vi "user_input.vi"() -> ()   [LabVIEW 2017]
uses:
  controls/AccountCmd.ctl
  controls/UpdateMessageCmd.ctl
  controls/UpdateMessageCtl.ctl
  controls/UserInputStateCmd.ctl
  controls/DisplayCommanda.ctl
  Downloads/ATM Simulator/Controls/DisplayControl.ctl
panel:
  out "queue 2":refnum<queue>
  in  "queue":refnum<queue>
  out "Parcel number":string
  in  "Phone number":string
  in  "Parcel number":string
  in  "User Input State":T1
  out "error out":errorcluster
  in  "error in (no error)":errorcluster
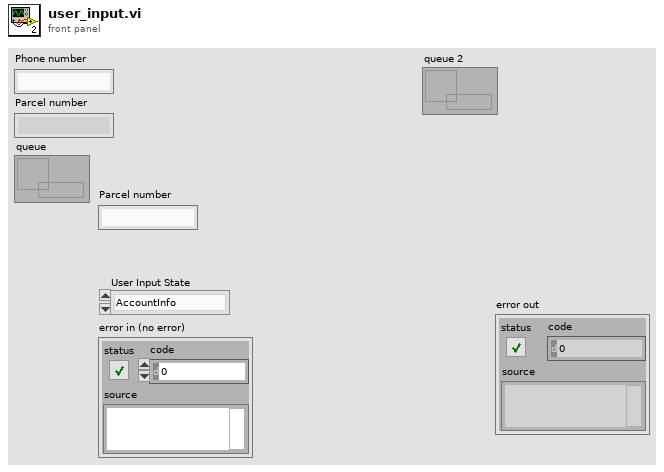
[diagram p1: front panel]
types:
  T1 = typedef "UserInputStateCmd.ctl" = enum16{"AccountInfo", "Withdrawal", "Deposit"}
  T2 = typedef "AccountCmd.ctl" = enum16{"Get parcel", "Get number", "Deposit", "Withdrawal"}
  T3 = typedef "UpdateMessageCtl.ctl" = cluster{"Command":T4, "Data":variant}
  T4 = typedef "UpdateMessageCmd.ctl" = enum16{"Welcome", "Main Menu", "Account Failed", "Session Terminated", "Deposit", "Deposit Complete", "Withdrawal", "Withdrawal Complete"}
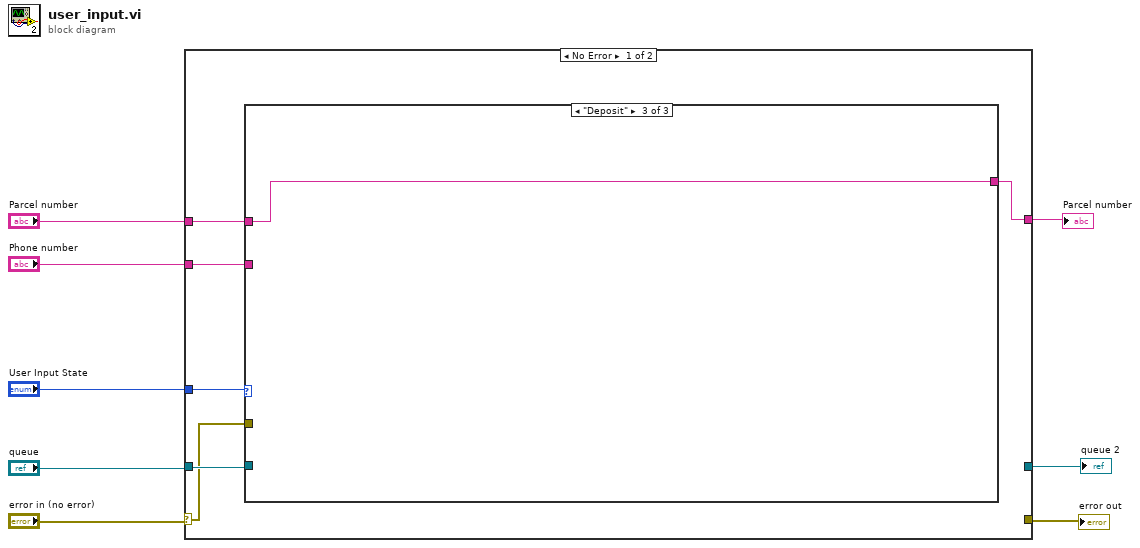
[diagram p0: block diagram]
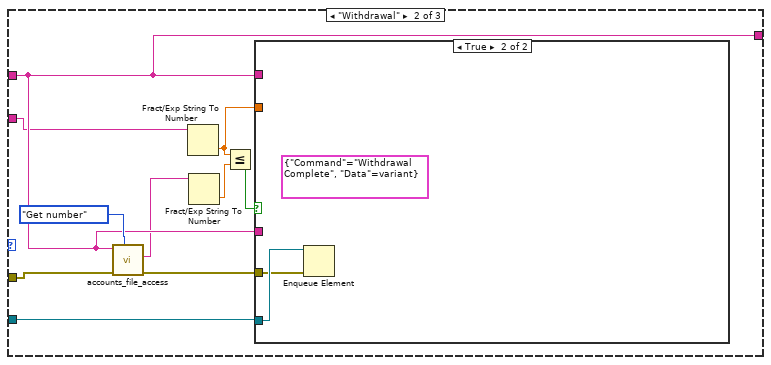
[diagram p3: hidden frame]
diagram:
  n1 = case shown="No Error" "error in (no error)" {
    selector: "error in (no error)" -> [w13 w31]
    tunnel: "queue" -> [w14 w30]
    tunnel: "User Input State" -> [w12 _]
    tunnel: "Parcel number" -> [w11 w29]
    tunnel: "Phone number" -> [w10 _]
    tunnel: [w9 w29] -> w3
    tunnel: [_ w31] -> w2
    tunnel: [_ w30] -> w1
    frame No Error {
      n2 = case shown="\"Deposit\"" w12 {
        tunnel: w14 -> [_ w25 _]
        tunnel: w13 -> [_ w22 _]
        tunnel: w11 -> [w15 w23 w28]
        tunnel: w10 -> [_ w19 _]
        tunnel: [w15 w23 w28] -> w9
        frame "AccountInfo", Default {
        }
        frame "Withdrawal" {
          n3 = call "accounts_file_access.vi"("AccountCommand"=AccountCmd."Get number", "error in (no error)"=w22, "Account"=w23) -> ("error out"=w21:errorcluster, "Value Out"=w20:string)  [unwired: 6 in]
          n4 = Fract/Exp String To Number(string=w19) -> (number=w18:dbl)  [unwired: 3 in, 1 out]
          n5 = Fract/Exp String To Number(string=w20) -> (number=w17:dbl)  [unwired: 3 in, 1 out]
          n6 = Less Or Equal?(x=w18, y=w17) -> (x <= y?=w16:bool)
          n7 = case shown="True" w16 {
            tunnel: w25 -> [_ w27]
            tunnel: w23 -> [_ _]
            tunnel: w23 -> [_ _]
            tunnel: w21 -> [_ w26]
            tunnel: w18 -> [_ _]
            frame False {
            }
            frame True {
              (unwired) T3 {"Command"=enum."Withdrawal Complete", "Data"=variant} ("Cluster")
              n8 = Enqueue Element(queue=w27, error in (no error)=w26) -> ()  [unwired: 2 in, 3 out]
            }
          }
        }
        frame "Deposit" {
        }
      }
    }
    frame Error {
    }
  }
  "Parcel number" <- w3
  "error out" <- w2
  "queue 2" <- w1
